vi "WSVCAP SHL Host TL RFFE Read.vi"(0 "Write Data In [DUT Ordered]":u8[][](array[numeric]) format="%02x", 7 "Socket Mask":u64=1 format="%02x", 11 "error in":errorcluster, 13 "Log (T)":bool=TRUE) -> (4 "Read Data Out":u8[][](array[numeric]) format="%.0x", 15 "error out":errorcluster)   [LabVIEW 2012]
uses:
  Type Defs/WSVCAP SHL Function Enum.ctl
panel:
  out "Status":u8[](array[numeric])
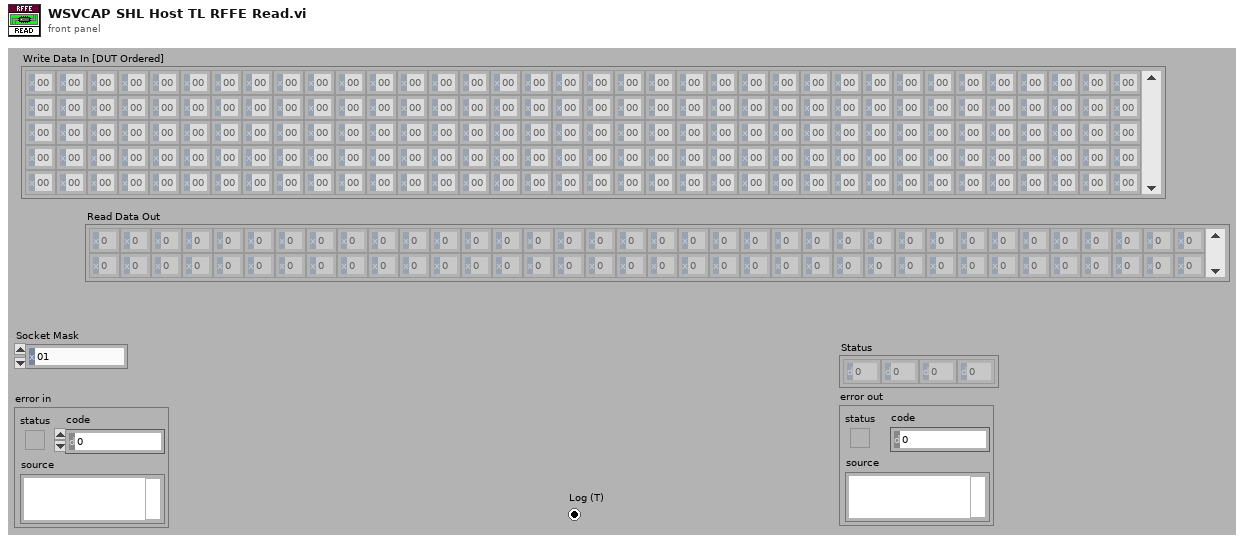
[diagram p1: front panel]
types:
  T1 = typedef "WSVCAP SHL Function Enum.ctl" = enum16{"Initialize", "Configure I2C", "Configure SPI", "Configure RFFE", "Write I2C", "Read I2C", "Write/Read SPI", "Start SPI Cycle", "Stop SPI Cycle", "Write RFFE", "Read RFFE", "Start RFFE Cycle", "Stop RFFE Cycle", "Get Status", "Close"}
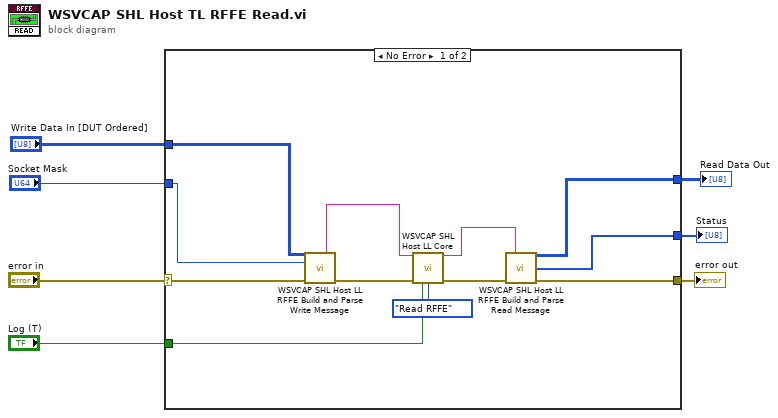
[diagram p0: block diagram]
diagram:
  n1 = case shown="No Error" "error in" {
    selector: "error in" -> [w12 w20]
    tunnel: [w16 w20] -> w7
    tunnel: "Socket Mask" -> [w10 _]
    tunnel: [w15 _] -> w4
    tunnel: [w14 _] -> w3
    tunnel: "Log (T)" -> [w13 _]
    tunnel: "Write Data In [DUT Ordered]" -> [w8 _]
    frame No Error {
      n2 = call "WSVCAP SHL Host LL RFFE Build and Parse Write Message.vi"("Write Data In [DUT Ordered]"=w8, "Socket Mask [U64] In"=w10, "error in"=w12) -> ("Message Out"=w9:string, "error out"=w11:errorcluster)  [unwired: 6 in, 5 out]
      n3 = call "WSVCAP SHL Host LL Core.vi"("Message In"=w9, "error in"=w11, "Log (T)"=w13, "Function"=WSVCAP_SHL_Function_Enum."Read RFFE") -> ("Message Out"=w17:string, "error out"=w18:errorcluster)  [unwired: 9 in, 1 out]
      n4 = call "WSVCAP SHL Host LL RFFE Build and Parse Read Message.vi"("Message In"=w17, "error in"=w18) -> ("Write Data Out"=w15:u8[][], "Status"=w14:u8[], "error out"=w16:errorcluster)  [unwired: 10 in, 1 out]
    }
    frame Error {
    }
  }
  "error out" <- w7
  "Read Data Out" <- w4
  "Status" <- w3
